vi "Connect.vi"(8 "error in (no error)":errorcluster, 11 "ESM303 in":refnum<class "ESM303.lvclass">) -> (0 "error out":errorcluster, 3 "ESM303 out":refnum<class "ESM303.lvclass">)   [LabVIEW 2018, in "ESM303.lvlib" / "ESM303.lvclass"]
uses:
  ESM303.lvclass
  <vilib>/Instr/_visa.llb/VISA Configure Serial Port (Instr).vi
  builds/Force Test Stand.lvlibp/Force Test Stand.lvclass
  C:/Users/Ron.Dexter.LUMINARTECH/Desktop/builds/Force Test Stand.lvlibp/Force Test Stand.lvclass
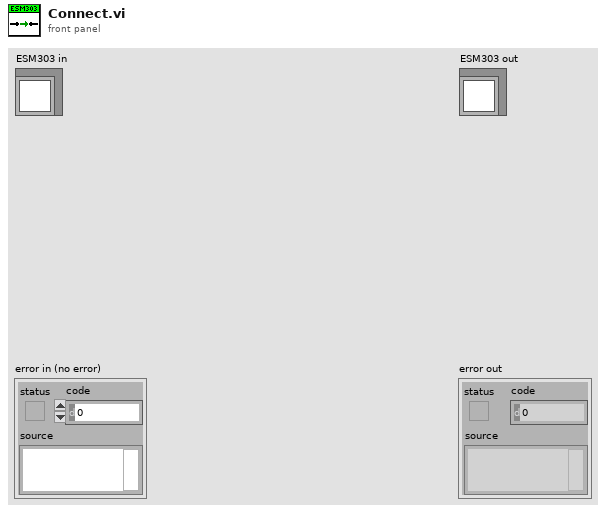
[diagram p1: front panel]
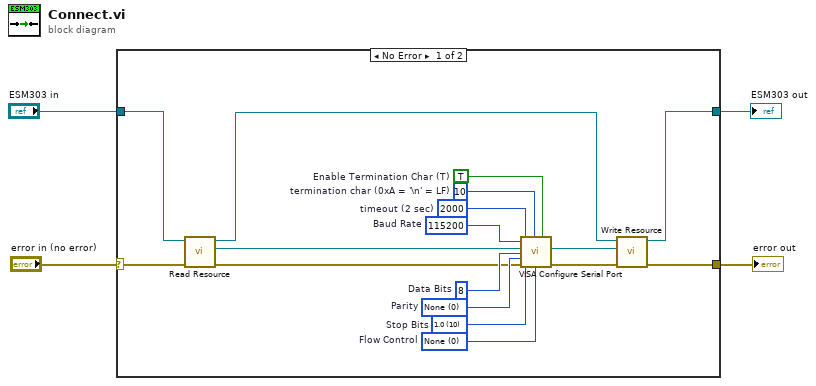
[diagram p0: block diagram]
diagram:
  n1 = case shown="No Error" "error in (no error)" {
    selector: "error in (no error)" -> [w20 w23]
    tunnel: [w19 w23] -> w3
    tunnel: [w18 w22] -> w2
    tunnel: "ESM303 in" -> [w21 w22]
    frame No Error {
      w10 = u32 115200  # Baud Rate
      w16 = u16 8  # Data Bits
      w11 = u16 0 items=["None", "Odd", "Even", "Mark", "Space"]  # Parity
      w14 = u16 10 items=["1.0"=10, "1.5"=15, "2.0"=20]  # Stop Bits
      w15 = u16 0 items=["None"=0, "XON/XOFF"=1, "RTS/CTS"=2, "DTR/DSR"=4]  # Flow Control
      w17 = u8 10  # termination char (0xA = '\n' = LF)
      w13 = TRUE  # Enable Termination Char (T)
      w12 = u32 2000  # timeout (2 sec)
      n2 = call "Read Resource.vi"("error in (no error)"=w20, "Force Test Stand in"=w21) -> ("error out"=w6:errorcluster, "Resource"=w9:refnum<visa-resource-name>, "Force Test Stand out"=w7:refnum<class "ESM303.lvclass">)  [unwired: 7 in]
      n3 = call-poly "VISA Configure Serial Port"("VISA resource name"=w9, "timeout (10sec)"=w12, "termination char\n(0xA = '\\n' = LF)"=w17, "Enable Termination\nChar (T)"=w13, "baud rate (9600)"=w10, "data bits (8)"=w16, "parity (0:none)"=w11, "error in (no error)"=w6, "stop bits (10: 1 bit)"=w14, "flow control (0:none)"=w15) -> ("VISA resource name out"=w5:refnum<visa-resource-name>, "error out"=w8:errorcluster)  [unwired: 4 in]
      n4 = call "Write Resource.vi"("error in (no error)"=w8, "Resource"=w5, "Force Test Stand in"=w7) -> ("error out"=w19:errorcluster, "Force Test Stand out"=w18:refnum<class "ESM303.lvclass">)  [unwired: 7 in]
    }
    frame Error {
    }
  }
  "error out" <- w3
  "ESM303 out" <- w2
